vi "Variaveis_Globais_CLP_Paralelo.vi"() -> ()   [LabVIEW 2019]
panel:
  in  "SPK-INV-001_ON_AUX 2":bool
  in  "SKS-NC-CV-006_AUX":bool
  in  "PC-TQ-ON":bool
  in  "PC-TQ-TD":dbl
  in  "PC-TQ-GP":dbl
  in  "PC-TQ-SP":dbl
  in  "PC-TQ-TI":dbl
  in  "SPW-INV-001_OFF_AUX":bool
  in  "SPK-INV-001_OFF_AUX":bool
  in  "SKM-FC-KF_AUX":dbl
  in  "SKM-FC-WF_AUX":dbl
  in  "SKM-PC-TQ_AUX":dbl
  in  "SKS-LC-K_AUX":dbl
  in  "SKS-LC-W_AUX":dbl
  in  "SKS-NC-CV-005_AUX":bool
  in  "SKS-NC-CV-004_AUX":bool
  in  "SPW-WR-VEL_AUX":dbl
  in  "SPW-RD-FLL_AUX":bool
  in  "SPW-RD-VVT_AUX":bool
  in  "SPW-RD-ALR_AUX":bool
  in  "SPK-WR-VEL_AUX":dbl
  in  "SPK-RD-FLL_AUX":bool
  in  "SPK-RD-VVT_AUX":bool
  in  "SPK-RD-ALR_AUX":bool
  in  "SKM-FC-AR_AUX":dbl
  in  "SKM-NC-CV-JMP_AUX":bool
  in  "SKM-NC-CV-COR_AUX":bool
  in  "SKM-NC-CV-LAM_AUX":bool
  in  "SPW-INV-001_ON_AUX":bool
  in  "SPW-NO-CV-008_AUX":bool
  in  "SPW-NO-CV-007_AUX":bool
  in  "SPW-NO-CV-006_AUX":bool
  in  "SPW-NO-CV-005_AUX":bool
  in  "SPW-NC-CV-004_AUX":bool
  in  "SPW-NC-CV-003_AUX":bool
  in  "SPW-NC-CV-002_AUX":bool
  in  "SPW-NC-CV-001_AUX":bool
  in  "SPK-INV-001_ON_AUX":bool
  in  "SKS-NC-CV-003_AUX":bool
  in  "SKS-NC-CV-002_AUX":bool
  in  "SKS-NC-CV-001_AUX":bool
  in  "SIW-NC-CV-002_AUX":bool
  in  "SIK-NC-CV-002_AUX":bool
  in  "SIT-NC-CV-001_AUX":bool
  in  "SIT-NC-CV-002_AUX":bool
  in  "SIK-NC-CV-001_AUX":bool
  in  "SIA-NC-CV-001_AUX":bool
  in  "SIW-NC-CV-001_AUX":bool
  in  "SPK-NO-CV-008_AUX":bool
  in  "SPK-NO-CV-007_AUX":bool
  in  "SPK-NO-CV-006_AUX":bool
  in  "SPK-NO-CV-005_AUX":bool
  in  "SPK-NC-CV-004_AUX":bool
  in  "SPK-NC-CV-003_AUX":bool
  in  "SPK-NC-CV-002_AUX":bool
  in  "SPK-NC-CV-001_AUX":bool
  # "SKID BOMBA"
  # "SKID DE MEDI敲O"
  # "SKID DE SEPARA敲O"
  # "SKID DE INJE敲O"
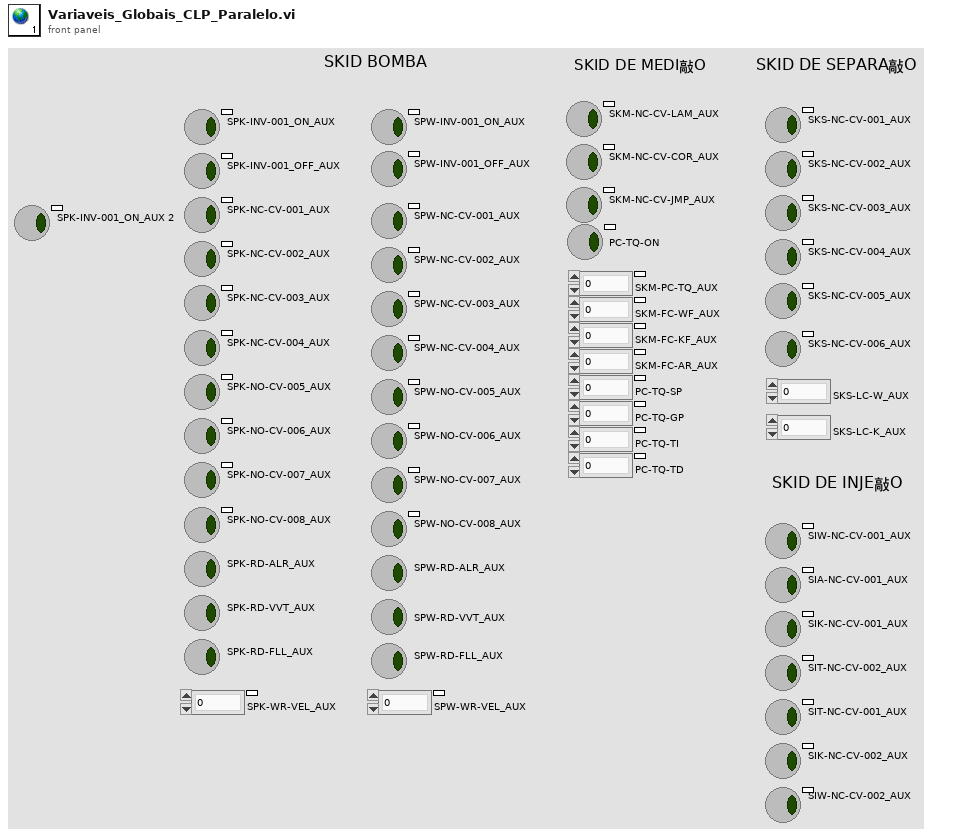
[diagram p1: front panel]
diagram:
